vi "XP2i.vi"(4 "error in":T13, 7 "Command":T14) -> (0 "error out":T13, 3 "Response":T11)   [LabVIEW 2018]
uses:
  MOKO_LabViewLibrary/MokoLowLevel/MokoLowLovelControl/MLLC_Command.ctl
  MOKO_LabViewLibrary/MokoLowLevel/MokoLowLovelControl/MLLC_Error.ctl
  MOKO_LabViewLibrary/MokoLowLevel/MokoLowLovelControl/MLLC_Mode.ctl
  MOKO_LabViewLibrary/MokoLowLevel/MokoLowLovelControl/MLLC_Response.ctl
  MOKO_LabViewLibrary/MokoLowLevel/MokoLowLovelControl/MLLC_DriverName.ctl
  MOKO_LabViewLibrary/MokoLowLevel/MokoLowLovelControl/MLLC_ResponseInit.ctl
  MOKO_LabViewLibrary/MokoLowLevel/MokoLowLovelControl/MLLC_Request.ctl
  MOKO_LabViewLibrary/MokoLowLevel/MokoLowLovelControl/MLLC_ErrorCode.ctl
  MOKO_LabViewLibrary/MokoLowLevel/MokoLowLovelControl/MLLC_ConnectCluster.ctl
  MOKO_LabViewLibrary/MokoLowLevel/MokoLowLovelControl/MLLC_InterfaceType.ctl
  MOKO_LabViewLibrary/MokoLowLevel/MokoLowLovelControl/MLLC_OpenedSession.ctl
  MOKO_LabViewLibrary/MokoLowLevel/MokoLowLovelControl/MLLC_InterfaceSettings.ctl
  MOKO_LabViewLibrary/MokoLowLevel/MokoLowLovelControl/MLLC_InterfaceKind.ctl
  MOKO_LabViewLibrary/MokoLowLevel/MokoLowLovelControl/MLLC_Rs232Settings.ctl
panel:
  in  "Settings":T6={"Saved Data"=variant, "Permanent data"={"Connect"={"InterfaceType"=enum."VISA", "OpenedSession"="COM4", "InterfaceSettings"={"Interface"=enum."RS232", "EOS 4 read"=enum."Default (=EOS 4 write)", "EOS 4 write"=enum."CR (\\r)", "TMO, ms"=2000, "Sett"=variant(cluster{"Baud Rate":u32, "Data Bits":u16, "Parity":u16, "Stop Bits":u16, "Flow Control":u16, "Eho":bool} {"Baud Rate"=75, "Data Bits"=0, "Parity"=0, "Stop Bits"=0, "Flow Control"=0, "Eho"=FALSE})}}}}
  in  "Error Code":T7=5420
  in  "Request":T8="?MOD"
  in  "ResponseInit":T9="XP2I"
  in  "Driver Name":T10="Crystal XP2"
  in  "Mode":T12=enum."Check"
  # "XP2i"
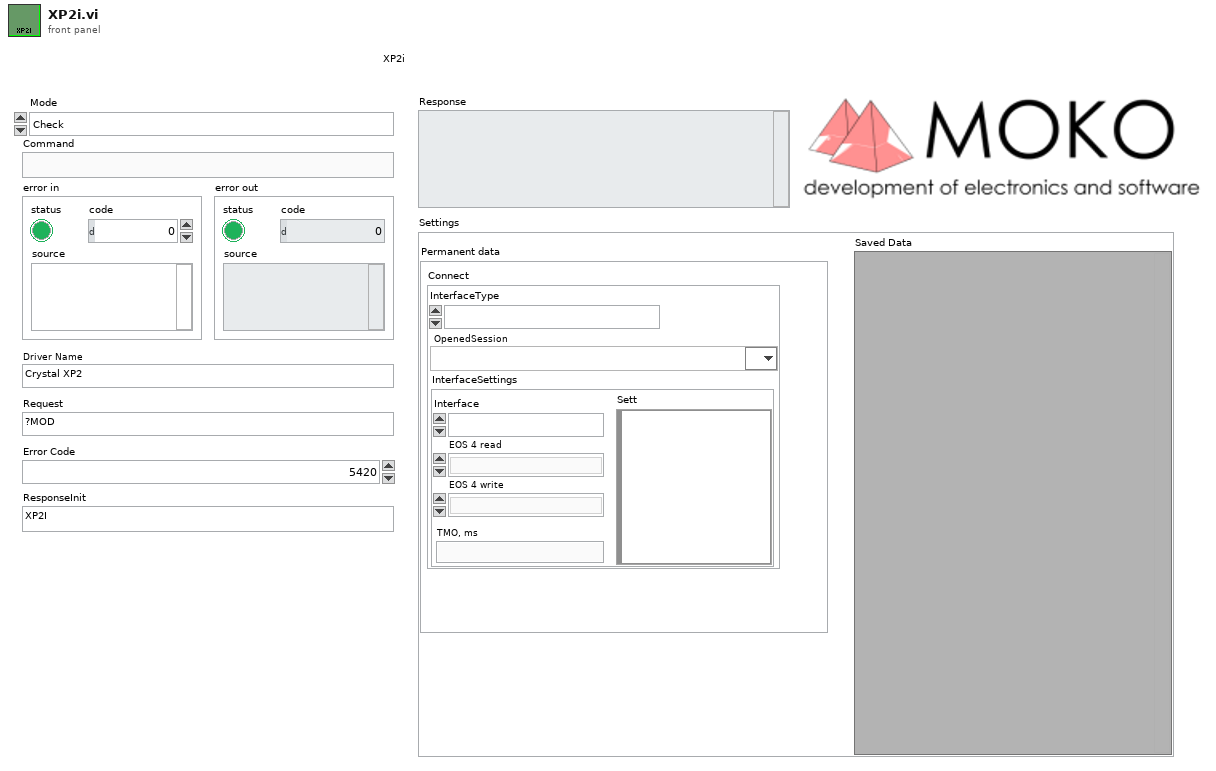
[diagram p1: front panel]
types:
  T1 = typedef "MLLC_ConnectCluster.ctl" = cluster{"InterfaceType":T2, "OpenedSession":T3, "InterfaceSettings":T4}
  T2 = typedef "MLLC_InterfaceType.ctl" = enum16{"VISA", "Prologix USB-GPIB"}
  T3 = typedef "MLLC_OpenedSession.ctl" = refnum<visa-resource-name>
  T4 = typedef "MLLC_InterfaceSettings.ctl" = cluster{"Interface":T5, "EOS 4 read":enum16{"Default (=EOS 4 write)", "CR (\\r)", "LF (\\n)", "None"}, "EOS 4 write":enum16{"CR+LF (\\r\\n)", "CR (\\r)", "LF (\\n)", "None"}, "TMO, ms":i32, "Sett":variant}
  T5 = typedef "MLLC_InterfaceKind.ctl" = enum16{"RS232", "GPIB", "USB", "Ethernet", "another"}
  T6 = cluster{"Saved Data":variant, "Permanent data":cluster{"Connect":T1}}
  T7 = typedef "MLLC_ErrorCode.ctl" = u32
  T8 = typedef "MLLC_Request.ctl" = string
  T9 = typedef "MLLC_ResponseInit.ctl" = string
  T10 = typedef "MLLC_DriverName.ctl" = string
  T11 = typedef "MLLC_Response.ctl" = string
  T12 = typedef "MLLC_Mode.ctl" = enum16{"get", "set", "close", "Init", "Check"}
  T13 = typedef "MLLC_Error.ctl" = errorcluster
  T14 = typedef "MLLC_Command.ctl" = string
  T15 = typedef "MLLC_Rs232Settings.ctl" = cluster{"Baud Rate":u32, "Data Bits":u16, "Parity":u16, "Stop Bits":u16, "Flow Control":u16, "Eho":bool, "Address":dbl}
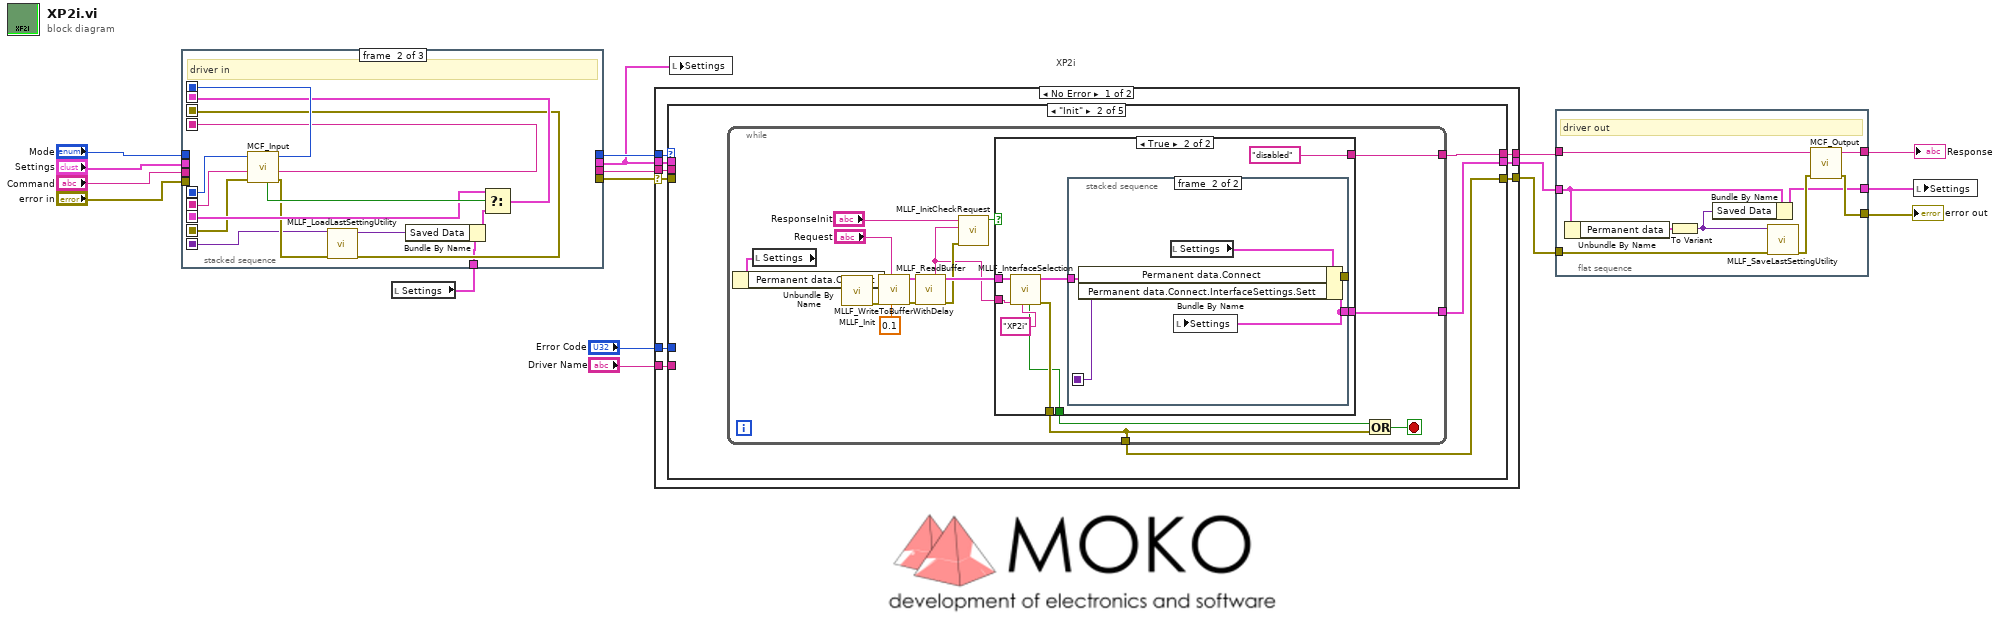
[diagram p0: block diagram]
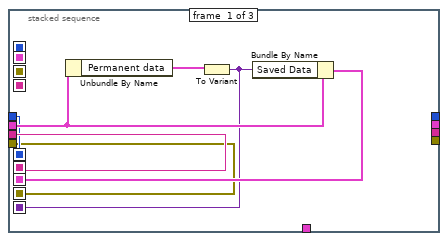
[diagram p2: hidden frame]
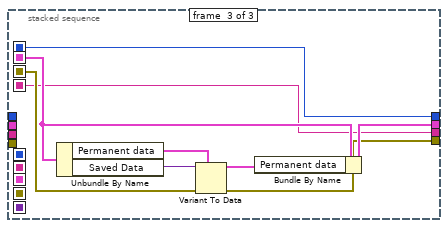
[diagram p3: hidden frame]
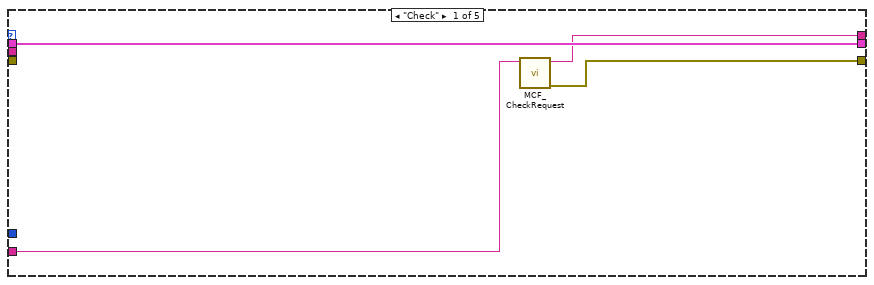
[diagram p4: hidden frame]
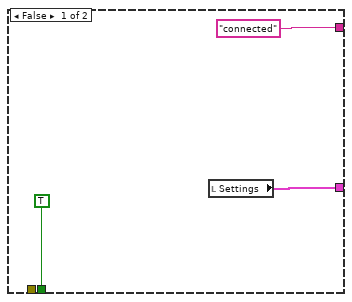
[diagram p5: hidden frame]
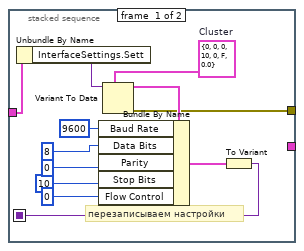
[diagram p6: hidden frame]
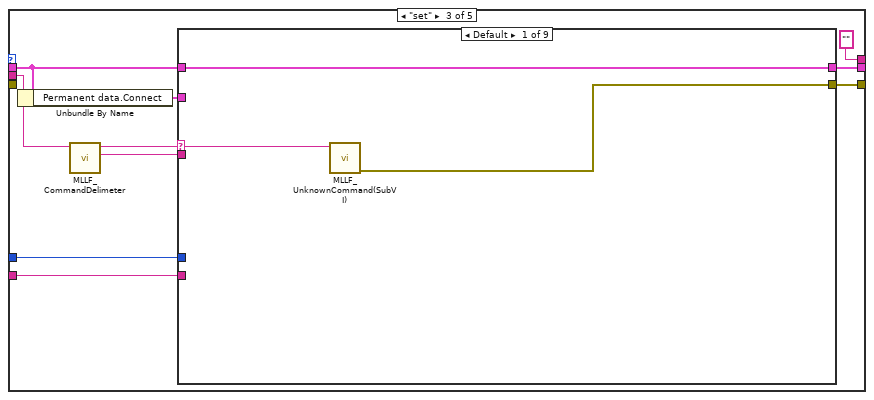
[diagram p7: hidden frame]
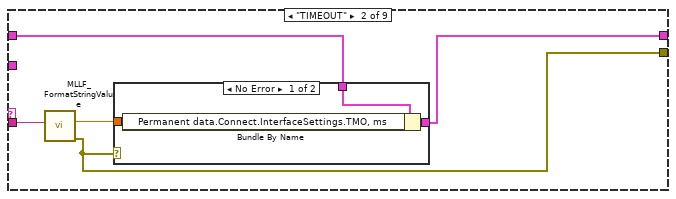
[diagram p8: hidden frame]
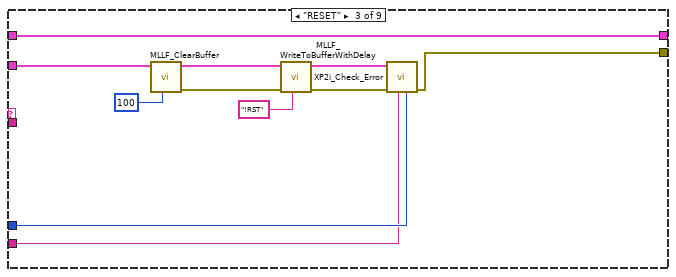
[diagram p10: hidden frame]
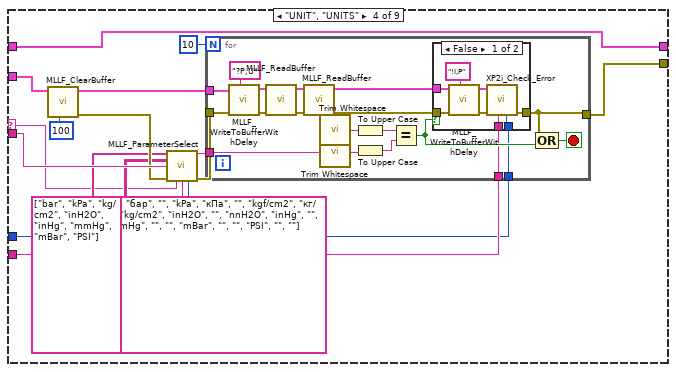
[diagram p11: hidden frame]
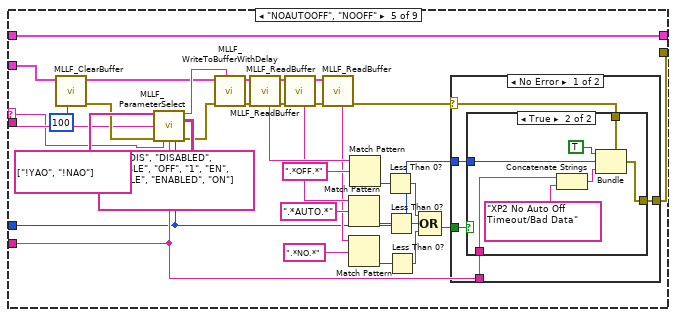
[diagram p13: hidden frame]
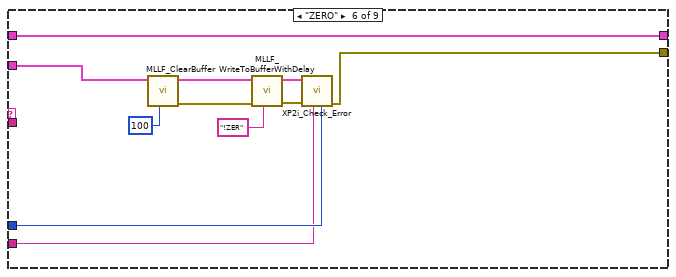
[diagram p16: hidden frame]
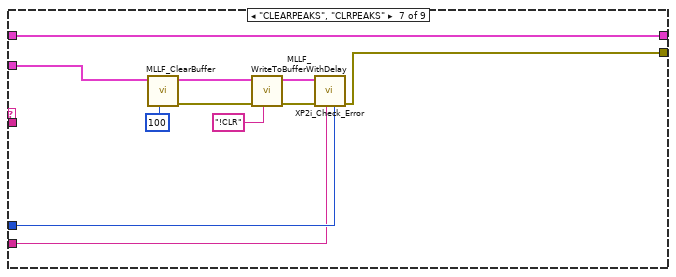
[diagram p17: hidden frame]
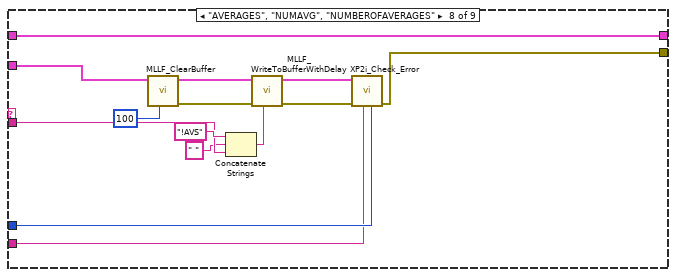
[diagram p18: hidden frame]
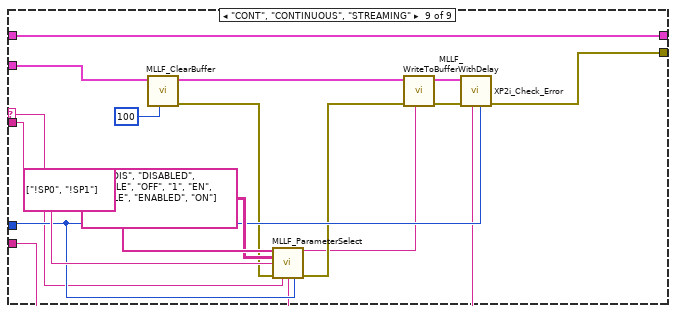
[diagram p19: hidden frame]
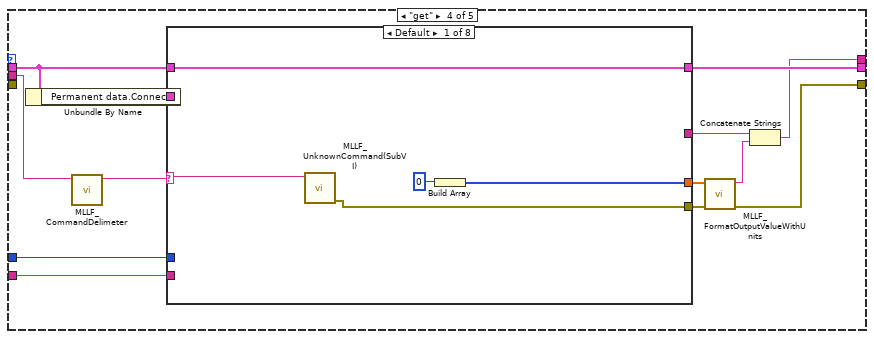
[diagram p20: hidden frame]
diagram:
  # "XP2i"
  n1 = local read "Settings"() -> (w7:T6)
  n2 = stacked-sequence {
    seq-local: [w20 _ _] -> [_ w36 _]
    seq-local: [w19 _ _] -> [_ w37 _]
    seq-local: [w22 _ _] -> [_ w32 _]
    seq-local: [w18 _ _] -> [_ w31 _]
    seq-local: [w21 _ _] -> [_ w27 _]
    seq-local: [_ w28 _] -> [_ _ w44]
    seq-local: [_ w38 _] -> [_ _ w41]
    seq-local: [_ w35 _] -> [_ _ w40]
    seq-local: [_ w34 _] -> [_ _ w45]
    tunnel: "Command" -> [w20 _ _]
    tunnel: "Mode" -> [w19 _ _]
    tunnel: "error in" -> [w18 _ _]
    tunnel: "Settings" -> [w23 _ _]
    tunnel: w7 -> [_ w26 _]
    tunnel: [_ _ w40] -> w9
    tunnel: [_ _ w43] -> w10
    tunnel: [_ _ w42] -> w8
    tunnel: [_ _ w41] -> w11
    frame #0 {
      n3 = Unbundle By Name(w23) -> ("Permanent data"=w24:cluster{"Connect":T1})
      n4 = To Variant(anything=w24) -> (Variant=w21:variant)
      n5 = Bundle By Name(cluster=w23, "Saved Data"=w21) -> (w22:T6)
    }
    frame #1 {
      # "driver in"
      n6 = call "MCF_Input.vi"("Error In"=w31, "Command in"=w36, "Mode in"=w37) -> ("Error Out"=w30:errorcluster, "Command out"=w35:string, "Mode out"=w38:T12, "Boolean"=w33:bool)  [unwired: 5 in]
      n7 = call "MLLF_LoadLastSettingUtility.vi"("Error In"=w30, "Save data in"=w27) -> ("Error Out"=w28:errorcluster, "Save data out"=w25:variant)  [unwired: 8 in]
      n8 = Bundle By Name(cluster=w26, "Saved Data"=w25) -> (w29:T6)
      n9 = Select(t=w32, s=w33, f=w29) -> (s? t:f=w34:T6)
    }
    frame #2 {
      n10 = Unbundle By Name(w45) -> ("Permanent data"=w46:cluster{"Connect":T1}, "Saved Data"=w39:variant)
      n11 = Variant To Data(error in=w44, type=w46, Variant=w39) -> (data=w47:cluster{"Connect":T1}, error out=w42:errorcluster)
      n12 = Bundle By Name(cluster=w45, "Permanent data"=w47) -> (w43:T6)
    }
  }
  n13 = case shown="No Error" w8 {
    selector: w8 -> [w53 w410]
    tunnel: [w48 w410] -> w4
    tunnel: w11 -> [w56 _]
    tunnel: [w55 _] -> w6
    tunnel: w9 -> [w54 _]
    tunnel: w10 -> [w50 w409]
    tunnel: "Error Code" -> [w52 _]
    tunnel: "Driver Name" -> [w51 _]
    tunnel: [w49 w409] -> w5
    frame No Error {
      n14 = case shown="\"Init\"" w56 {
        tunnel: [w58 w63 "" ("Output String") w294 "" ("Output String")] -> w55
        tunnel: w54 -> [_ _ w111 w287 _]
        tunnel: w53 -> [_ _ _ _ _]
        tunnel: w52 -> [_ _ w118 w297 _]
        tunnel: w51 -> [w59 _ w115 w296 _]
        tunnel: w50 -> [w60 _ w117 w298 w407]
        tunnel: [w60 w62 w116 w295 w407] -> w49
        tunnel: [w57 w61 w114 w288 w406] -> w48
        frame "Check" {
          n15 = call "MCF_CheckRequest.vi"("Driver Name"=w59) -> ("Error Out"=w57:errorcluster, "Output String"=w58:string)  [unwired: 9 in]
        }
        frame "Init" {
          n16 = while {
            tunnel: [w76] -> w61
            tunnel: [w73] -> w63
            tunnel: [w72] -> w62
            stop <- w78 stop-if-true
            n17 = local read "Settings"() -> (w67:T6)
            n18 = Unbundle By Name(w67) -> ("Permanent data.Connect"=w66:T1)
            n19 = call "MLLF_Init.vi"("DriverConnect in"=w66) -> ("Error Out"=w80:errorcluster, "DriverConnect out"=w79:T1)  [unwired: 7 in]
            n20 = call "MLLF_WriteToBufferWithDelay.vi"("Delay Time ( 0,05 s)"=0.1 ("Delay Time (s)"), "Command"="Request", "Error In"=w80, "DriverConnect in"=w79) -> ("Error Out"=w75:errorcluster, "DriverConnect out"=w65:T1)  [unwired: 6 in]
            n21 = call "MLLF_ReadBuffer.vi"("Error In"=w75, "DriverConnect in"=w65) -> ("Error Out"=w71:errorcluster, "DriverConnect out"=w81:T1, "String"=w64:string)  [unwired: 6 in]
            n22 = call "MLLF_InitCheckRequest.vi"("error in (no error)"=w71, "Answer"=w64, "Response Init"="ResponseInit") -> ("Design"=w70:bool)  [unwired: 5 in, 3 out]
            n23 = case shown="True" w70 {
              tunnel: w81 -> [_ w91]
              tunnel: [TRUE w87] -> w77
              tunnel: [_ w92] -> w76
              tunnel: ["connected" "disabled"] -> w73
              tunnel: [w82 w86] -> w72
              tunnel: w64 -> [_ w85]
              frame False {
                n24 = local read "Settings"() -> (w82:T6)
              }
              frame True {
                n25 = call "MLLF_InterfaceSelection.vi"("Driver Name"="XP2i" ("String"), "Answer:"=w85, "DriverConnect in"=w91) -> ("error out"=w92:T13, "DriverConnect out"=w90:T1, "stop init?"=w87:bool)  [unwired: 4 in, 2 out]
                n26 = stacked-sequence {
                  seq-local: [w96 _] -> [_ w105]
                  tunnel: w90 -> [w94 w106]
                  tunnel: [w97 _] -> _
                  tunnel: [_ w107] -> w86
                  frame #0 {
                    w98 = T15 {"Baud Rate"=0, "Data Bits"=0, "Parity"=0, "Stop Bits"=10, "Flow Control"=0, "Eho"=FALSE, "Address"=0.0}  # Cluster
                    # "перезаписываем настройки"
                    n27 = Unbundle By Name(w94) -> ("InterfaceSettings.Sett"=w93:variant)
                    n28 = Variant To Data(type=w98, Variant=w93) -> (data=w99:T15, error out=w97:errorcluster)  [unwired: 1 in]
                    n29 = Bundle By Name(cluster=w99, "Baud Rate"=u32 9600, "Data Bits"=u16 8 ("Serial Settings:Data Bits"), "Parity"=u16 0 ("Serial Settings:Parity"), "Stop Bits"=u16 10 ("Serial Settings:Stop Bits"), "Flow Control"=u16 0 ("Serial Settings:Flow Control")) -> (w104:T15)
                    n30 = To Variant(anything=w104) -> (Variant=w96:variant)
                  }
                  frame #1 {
                    n31 = local read "Settings"() -> (w108:T6)
                    n32 = Bundle By Name(cluster=w108, "Permanent data.Connect"=w106, "Permanent data.Connect.InterfaceSettings.Sett"=w105) -> (w107:T6)
                    n33 = local write "Settings"(w107) -> ()
                  }
                }
              }
            }
            n34 = Or(x=w77, y=w76) -> (x .or. y?=w78:bool)
          }
        }
        frame "set" {
          n35 = Unbundle By Name(w117) -> ("Permanent data.Connect"=w112:T1)
          n36 = call "MLLF_CommandDelimeter.vi"("command with param"=w111) -> ("param 1"=w109:string, "command"=w110:string)  [unwired: 6 in, 3 out]
          n37 = case shown="Default" w110 {
            selector: w110 -> [w120 _ _ w142 w186 _ _ _ w271]
            tunnel: w109 -> [_ w124 _ w154 w194 _ _ w261 w280]
            tunnel: w118 -> [_ _ w139 w152 w196 w239 w250 w265 w279]
            tunnel: w117 -> [w121 w125 w141 w145 w219 w244 w255 w269 w285]
            tunnel: [w121 w126 w141 w145 w219 w244 w255 w269 w285] -> w116
            tunnel: w115 -> [_ _ w138 w153 w197 w238 w249 w264 w270]
            tunnel: w112 -> [_ _ w132 w144 w188 w235 w246 w257 w273]
            tunnel: [w119 w122 w131 w143 w187 w234 w245 w256 w272] -> w114
            frame Default {
              n38 = call "MLLF_UnknownCommand(SubVI).vi"("Unknown command"=w120) -> ("error out"=w119:errorcluster)  [unwired: 10 in]
            }
            frame "TIMEOUT" {
              n39 = call "MLLF_FormatStringValue.vi"("String Value"=w124) -> ("error out"=w122:T13, "number"=w123:dbl)  [unwired: 8 in, 1 out]
              n40 = case shown="No Error" w122 {
                tunnel: [w129 w130] -> w126
                tunnel: w125 -> [w128 w130]
                tunnel: w123 -> [w127 _]
                frame No Error {
                  n41 = Bundle By Name(cluster=w128, "Permanent data.Connect.InterfaceSettings.TMO, ms"=w127) -> (w129:T6)
                }
                frame Error {
                }
              }
            }
            frame "RESET" {
              n42 = call "MLLF_ClearBuffer.vi"("Timeout(default = 300 ms)"=u32 100 ("Timeout"), "DriverConnect in"=w132) -> ("Error Out"=w136:errorcluster, "DriverConnect out"=w135:T1)  [unwired: 6 in, 1 out]
              n43 = call "MLLF_WriteToBufferWithDelay.vi"("Command"="!RST" ("String"), "Error In"=w136, "DriverConnect in"=w135) -> ("Error Out"=w134:errorcluster, "DriverConnect out"=w140:T1)  [unwired: 7 in]
              n44 = call "XP2i_Check_Error.vi"("Error Code"=w139, "Driver Name"=w138, "Error In"=w134, "DriverConnect in"=w140) -> ("Error Out"=w131:errorcluster)  [unwired: 6 in, 1 out]
            }
            frame "UNIT", "UNITS" {
              n45 = call "MLLF_ClearBuffer.vi"("Timeout(default = 300 ms)"=u32 100 ("Timeout"), "DriverConnect in"=w144) -> ("Error Out"=w151:errorcluster, "DriverConnect out"=w155:T1)  [unwired: 6 in, 1 out]
              n46 = call "MLLF_ParameterSelect.vi"("Command to equipment"=string[] ["bar", "kPa", "kg/cm2", "inH2O", "inHg", "mmHg", "mBar", "PSI"] ("Parameters 2 equipment"), "Names"=string[][] [["bar", "бар", ""], ["kPa", "кПа", ""], ["kgf/cm2", "кг/см2", "kg/cm2"], ["inH2O", "", "nnH2O"], ["inHg", "", ""], ["mmHg", "", ""], ["mBar", "", ""], ["PSI", "", ""]], "Input"=w154, "Error In"=w151, "Command"=w142, "Driver Name"=w153, "Error Code"=w152) -> ("Choice"=w149:string, "Error Out"=w150:errorcluster)  [unwired: 7 in]
              n47 = for {
                N: 10 -> [_]
                tunnel: w155 -> [w166]
                tunnel: [w160] -> w143
                tunnel: w149 -> [w164]
                tunnel: w153 -> [w158]
                tunnel: w152 -> [w157]
                tunnel: w150 -> [w165]
                stop <- w172 stop-if-true
                n48 = call "MLLF_WriteToBufferWithDelay.vi"("Command"="?P,U" ("String"), "Error In"=w165, "DriverConnect in"=w166) -> ("Error Out"=w168:errorcluster, "DriverConnect out"=w175:T1)  [unwired: 7 in]
                n49 = call "MLLF_ReadBuffer.vi"("Error In"=w168, "DriverConnect in"=w175) -> ("Error Out"=w171:errorcluster, "DriverConnect out"=w170:T1)  [unwired: 6 in, 1 out]
                n50 = call "MLLF_ReadBuffer.vi"("Error In"=w171, "DriverConnect in"=w170) -> ("Error Out"=w161:errorcluster, "DriverConnect out"=w162:T1, "String"=w169:string)  [unwired: 6 in]
                n51 = call <vilib>:"Trim Whitespace.vi"("string"=w169) -> ("trimmed string"=w167:string)  [unwired: 1 in]
                n52 = call <vilib>:"Trim Whitespace.vi"("string"=w164) -> ("trimmed string"=w163:string)  [unwired: 1 in]
                n53 = To Upper Case(1:w167) -> (0:w174:string)
                n54 = To Upper Case(1:w163) -> (0:w173:string)
                n55 = Equal?(x=w174, y=w173) -> (x = y?=w159:bool)
                n56 = case shown="False" w159 {
                  tunnel: w162 -> [w181 _]
                  tunnel: w161 -> [w180 w185]
                  tunnel: [w179 w185] -> w160
                  tunnel: w158 -> [w178 _]
                  tunnel: w157 -> [w177 _]
                  frame False {
                    n57 = call "MLLF_WriteToBufferWithDelay.vi"("Command"="!I,P" ("String"), "Error In"=w180, "DriverConnect in"=w181) -> ("Error Out"=w182:errorcluster, "DriverConnect out"=w183:T1)  [unwired: 7 in]
                    n58 = call "XP2i_Check_Error.vi"("Error Code"=w177, "Driver Name"=w178, "Error In"=w182, "DriverConnect in"=w183) -> ("Error Out"=w179:errorcluster)  [unwired: 6 in, 1 out]
                  }
                  frame True {
                  }
                }
                n59 = Compound Arithmetic op=OR(w160, w159) -> (w172:bool)
              }
            }
            frame "NOAUTOOFF", "NOOFF" {
              n60 = call "MLLF_ClearBuffer.vi"("Timeout(default = 300 ms)"=u32 100 ("Timeout"), "DriverConnect in"=w188) -> ("Error Out"=w195:errorcluster, "DriverConnect out"=w191:T1)  [unwired: 6 in, 1 out]
              n61 = call "MLLF_ParameterSelect.vi"("Command to equipment"=string[] ["!YAO", "!NAO"] ("Names"), "Names"=string[][] [["0", "DIS", "DISABLED", "DISABLE", "OFF"], ["1", "EN", "ENABLE", "ENABLED", "ON"]], "Input"=w194, "Error In"=w195, "Command"=w186, "Driver Name"=w197, "Error Code"=w196) -> ("Choice"=w193:string, "Error Out"=w192:errorcluster)  [unwired: 7 in]
              n62 = call "MLLF_WriteToBufferWithDelay.vi"("Command"=w193, "Error In"=w192, "DriverConnect in"=w191) -> ("Error Out"=w189:errorcluster, "DriverConnect out"=w218:T1)  [unwired: 7 in]
              n63 = call "MLLF_ReadBuffer.vi"("Error In"=w189, "DriverConnect in"=w218) -> ("Error Out"=w217:errorcluster, "DriverConnect out"=w216:T1, "String"=w204:string)  [unwired: 6 in]
              n64 = call "MLLF_ReadBuffer.vi"("Error In"=w217, "DriverConnect in"=w216) -> ("Error Out"=w215:errorcluster, "DriverConnect out"=w214:T1, "String"=w203:string)  [unwired: 6 in]
              n65 = call "MLLF_ReadBuffer.vi"("Error In"=w215, "DriverConnect in"=w214) -> ("Error Out"=w201:errorcluster, "String"=w202:string)  [unwired: 6 in, 1 out]
              n66 = Match Pattern(string=w203, regular expression=".*AUTO.*") -> (offset past match=w209:i32)  [unwired: 1 in, 3 out]
              n67 = Match Pattern(string=w202, regular expression=".*NO.*") -> (offset past match=w210:i32)  [unwired: 1 in, 3 out]
              n68 = Match Pattern(string=w204, regular expression=".*OFF.*") -> (offset past match=w208:i32)  [unwired: 1 in, 3 out]
              n69 = Less Than 0?(x=w208) -> (x < 0?=w211:bool)
              n70 = Less Than 0?(x=w209) -> (x < 0?=w212:bool)
              n71 = Less Than 0?(x=w210) -> (x < 0?=w213:bool)
              n72 = Compound Arithmetic op=OR(w211, w212, w213) -> (w200:bool)
              n73 = case shown="No Error" w201 {
                selector: w201 -> [w220 w233]
                tunnel: [w224 w233] -> w187
                tunnel: w200 -> [w223 _]
                tunnel: w196 -> [w222 _]
                tunnel: w197 -> [w221 _]
                frame No Error {
                  n74 = case shown="True" w223 {
                    tunnel: [w225 w231] -> w224
                    tunnel: w222 -> [_ w230]
                    tunnel: w221 -> [_ w228]
                    tunnel: w220 -> [w225 w226]
                    frame False {
                    }
                    frame True {
                      n75 = Concatenate Strings(w228, "XP2 No Auto Off Timeout/Bad Data") -> (w227:string)
                      n76 = Bundle(cluster=w226, "status"=TRUE, "code"=w230, "source"=w227) -> (w231:errorcluster)
                    }
                  }
                }
                frame Error {
                }
              }
            }
            frame "ZERO" {
              n77 = call "MLLF_ClearBuffer.vi"("Timeout(default = 300 ms)"=u32 100 ("Timeout"), "DriverConnect in"=w235) -> ("Error Out"=w242:errorcluster, "DriverConnect out"=w241:T1)  [unwired: 6 in, 1 out]
              n78 = call "MLLF_WriteToBufferWithDelay.vi"("Command"="!ZER" ("String"), "Error In"=w242, "DriverConnect in"=w241) -> ("Error Out"=w236:errorcluster, "DriverConnect out"=w240:T1)  [unwired: 7 in]
              n79 = call "XP2i_Check_Error.vi"("Error Code"=w239, "Driver Name"=w238, "Error In"=w236, "DriverConnect in"=w240) -> ("Error Out"=w234:errorcluster)  [unwired: 6 in, 1 out]
            }
            frame "CLEARPEAKS", "CLRPEAKS" {
              n80 = call "MLLF_ClearBuffer.vi"("Timeout(default = 300 ms)"=u32 100 ("Timeout"), "DriverConnect in"=w246) -> ("Error Out"=w253:errorcluster, "DriverConnect out"=w252:T1)  [unwired: 6 in, 1 out]
              n81 = call "MLLF_WriteToBufferWithDelay.vi"("Command"="!CLR" ("String"), "Error In"=w253, "DriverConnect in"=w252) -> ("Error Out"=w248:errorcluster, "DriverConnect out"=w251:T1)  [unwired: 7 in]
              n82 = call "XP2i_Check_Error.vi"("Error Code"=w250, "Driver Name"=w249, "Error In"=w248, "DriverConnect in"=w251) -> ("Error Out"=w245:errorcluster)  [unwired: 6 in, 1 out]
            }
            frame "AVERAGES", "NUMAVG", "NUMBEROFAVERAGES" {
              n83 = call "MLLF_ClearBuffer.vi"("Timeout(default = 300 ms)"=u32 100 ("Timeout"), "DriverConnect in"=w257) -> ("Error Out"=w268:errorcluster, "DriverConnect out"=w267:T1)  [unwired: 6 in, 1 out]
              n84 = Concatenate Strings("!AVS" ("String"), " " ("string"), w261) -> (w262:string)
              n85 = call "MLLF_WriteToBufferWithDelay.vi"("Command"=w262, "Error In"=w268, "DriverConnect in"=w267) -> ("Error Out"=w259:errorcluster, "DriverConnect out"=w266:T1)  [unwired: 7 in]
              n86 = call "XP2i_Check_Error.vi"("Error Code"=w265, "Driver Name"=w264, "Error In"=w259, "DriverConnect in"=w266) -> ("Error Out"=w256:errorcluster)  [unwired: 6 in, 1 out]
            }
            frame "CONT", "CONTINUOUS", "STREAMING" {
              n87 = call "MLLF_ClearBuffer.vi"("Timeout(default = 300 ms)"=u32 100 ("Timeout"), "DriverConnect in"=w273) -> ("Error Out"=w278:errorcluster, "DriverConnect out"=w284:T1)  [unwired: 6 in, 1 out]
              n88 = call "MLLF_ParameterSelect.vi"("Command to equipment"=string[] ["!SP0", "!SP1"] ("Names"), "Names"=string[][] [["0", "DIS", "DISABLED", "DISABLE", "OFF"], ["1", "EN", "ENABLE", "ENABLED", "ON"]], "Input"=w280, "Error In"=w278, "Command"=w271, "Driver Name"=w270, "Error Code"=w279) -> ("Choice"=w276:string, "Error Out"=w277:errorcluster)  [unwired: 7 in]
              n89 = call "MLLF_WriteToBufferWithDelay.vi"("Command"=w276, "Error In"=w277, "DriverConnect in"=w284) -> ("Error Out"=w275:errorcluster, "DriverConnect out"=w283:T1)  [unwired: 7 in]
              n90 = call "XP2i_Check_Error.vi"("Error Code"=w279, "Driver Name"=w270, "Error In"=w275, "DriverConnect in"=w283) -> ("Error Out"=w272:errorcluster)  [unwired: 6 in, 1 out]
            }
          }
        }
        frame "get" {
          n91 = Unbundle By Name(w298) -> ("Permanent data.Connect"=w289:T1)
          n92 = call "MLLF_CommandDelimeter.vi"("command with param"=w287) -> ("command"=w286:string)  [unwired: 6 in, 4 out]
          n93 = case shown="Default" w286 {
            selector: w286 -> [w300 _ _ _ _ _ _ _]
            tunnel: [w299 _ w315 w329 w346 w363 w380 w397] -> w293
            tunnel: w297 -> [_ _ _ _ _ _ _ _]
            tunnel: [w303 w306 w319 w336 w353 w370 w387 w404] -> w295
            tunnel: w298 -> [w303 w306 w319 w336 w353 w370 w387 w404]
            tunnel: [w301 w304 _ w333 w350 w367 w384 w401] -> w292
            tunnel: w296 -> [_ _ _ _ _ _ _ _]
            tunnel: [_ _ w310 _ _ _ _ _] -> w290
            tunnel: w289 -> [_ _ w307 w320 w337 w354 w371 w388]
            frame Default {
              n94 = call "MLLF_UnknownCommand(SubVI).vi"("Unknown command"=w300) -> ("error out"=w299:errorcluster)  [unwired: 10 in]
              n95 = Build Array(0 ("TimeOut")) -> (w301:i32[])
            }
            frame "TIMEOUT" {
              n96 = Unbundle By Name(w306) -> ("Permanent data.Connect.InterfaceSettings.TMO, ms"=w305:i32)
              n97 = Build Array(w305) -> (w304:i32[])
            }
            frame "PRESSURE" {
              n98 = call "MLLF_ClearBuffer.vi"("Timeout(default = 300 ms)"=u32 100 ("Timeout"), "DriverConnect in"=w307) -> ("Error Out"=w316:errorcluster, "DriverConnect out"=w317:T1)  [unwired: 6 in, 1 out]
              n99 = call "MLLF_WriteToBufferWithDelay.vi"("Command"="?PRE" ("String"), "Error In"=w316, "DriverConnect in"=w317) -> ("Error Out"=w309:errorcluster, "DriverConnect out"=w314:T1)  [unwired: 7 in]
              n100 = call "MLLF_ReadBuffer.vi"("Error In"=w309, "DriverConnect in"=w314) -> ("Error Out"=w315:errorcluster, "String"=w313:string)  [unwired: 6 in, 1 out]
              n101 = Match Pattern(string=w313, regular expression=",") -> (before substring=w311:string)  [unwired: 1 in, 3 out]
              n102 = call <vilib>:"Trim Whitespace.vi"("string"=w311) -> ("trimmed string"=w310:string)  [unwired: 1 in]
            }
            frame "PRESSUREHIGH" {
              n103 = call "MLLF_ClearBuffer.vi"("Timeout(default = 300 ms)"=u32 100 ("Timeout"), "DriverConnect in"=w320) -> ("Error Out"=w330:errorcluster, "DriverConnect out"=w331:T1)  [unwired: 6 in, 1 out]
              n104 = call "MLLF_WriteToBufferWithDelay.vi"("Command"="?P,H" ("String"), "Error In"=w330, "DriverConnect in"=w331) -> ("Error Out"=w322:errorcluster, "DriverConnect out"=w326:T1)  [unwired: 7 in]
              n105 = call "MLLF_ReadBuffer.vi"("Error In"=w322, "DriverConnect in"=w326) -> ("Error Out"=w325:errorcluster, "DriverConnect out"=w324:T1, "String"=w323:string)  [unwired: 6 in]
              n106 = call "MLLF_ReadBuffer.vi"("Error In"=w325, "DriverConnect in"=w324) -> ("Error Out"=w329:errorcluster)  [unwired: 6 in, 2 out]
              n107 = Match Pattern(string=w323, regular expression=",") -> (before substring=w327:string)  [unwired: 1 in, 3 out]
              n108 = Fract/Exp String To Number(use system decimal point (T)=FALSE, string=w327) -> (number=w334:dbl)  [unwired: 2 in, 1 out]
              n109 = Build Array(w334) -> (w333:dbl[])
            }
            frame "PRESSURELOW" {
              n110 = call "MLLF_ClearBuffer.vi"("Timeout(default = 300 ms)"=u32 100 ("Timeout"), "DriverConnect in"=w337) -> ("Error Out"=w347:errorcluster, "DriverConnect out"=w348:T1)  [unwired: 6 in, 1 out]
              n111 = call "MLLF_WriteToBufferWithDelay.vi"("Command"="?P,L" ("String"), "Error In"=w347, "DriverConnect in"=w348) -> ("Error Out"=w339:errorcluster, "DriverConnect out"=w343:T1)  [unwired: 7 in]
              n112 = call "MLLF_ReadBuffer.vi"("Error In"=w339, "DriverConnect in"=w343) -> ("Error Out"=w342:errorcluster, "DriverConnect out"=w341:T1, "String"=w340:string)  [unwired: 6 in]
              n113 = call "MLLF_ReadBuffer.vi"("Error In"=w342, "DriverConnect in"=w341) -> ("Error Out"=w346:errorcluster)  [unwired: 6 in, 2 out]
              n114 = Match Pattern(string=w340, regular expression=",") -> (before substring=w344:string)  [unwired: 1 in, 3 out]
              n115 = Fract/Exp String To Number(use system decimal point (T)=FALSE, string=w344) -> (number=w351:dbl)  [unwired: 2 in, 1 out]
              n116 = Build Array(w351) -> (w350:dbl[])
            }
            frame "AVERAGEPRESSURE", "AVGPRESS", "AVGPRESSURE" {
              n117 = call "MLLF_ClearBuffer.vi"("Timeout(default = 300 ms)"=u32 100 ("Timeout"), "DriverConnect in"=w354) -> ("Error Out"=w364:errorcluster, "DriverConnect out"=w365:T1)  [unwired: 6 in, 1 out]
              n118 = call "MLLF_WriteToBufferWithDelay.vi"("Command"="?P,A" ("String"), "Error In"=w364, "DriverConnect in"=w365) -> ("Error Out"=w356:errorcluster, "DriverConnect out"=w360:T1)  [unwired: 7 in]
              n119 = call "MLLF_ReadBuffer.vi"("Error In"=w356, "DriverConnect in"=w360) -> ("Error Out"=w359:errorcluster, "DriverConnect out"=w358:T1, "String"=w357:string)  [unwired: 6 in]
              n120 = call "MLLF_ReadBuffer.vi"("Error In"=w359, "DriverConnect in"=w358) -> ("Error Out"=w363:errorcluster)  [unwired: 6 in, 2 out]
              n121 = Match Pattern(string=w357, regular expression=",") -> (before substring=w361:string)  [unwired: 1 in, 3 out]
              n122 = Fract/Exp String To Number(use system decimal point (T)=FALSE, string=w361) -> (number=w368:dbl)  [unwired: 2 in, 1 out]
              n123 = Build Array(w368) -> (w367:dbl[])
            }
            frame "RANGE" {
              n124 = call "MLLF_ClearBuffer.vi"("Timeout(default = 300 ms)"=u32 100 ("Timeout"), "DriverConnect in"=w371) -> ("Error Out"=w381:errorcluster, "DriverConnect out"=w382:T1)  [unwired: 6 in, 1 out]
              n125 = call "MLLF_WriteToBufferWithDelay.vi"("Command"="?RNG" ("String"), "Error In"=w381, "DriverConnect in"=w382) -> ("Error Out"=w373:errorcluster, "DriverConnect out"=w377:T1)  [unwired: 7 in]
              n126 = call "MLLF_ReadBuffer.vi"("Error In"=w373, "DriverConnect in"=w377) -> ("Error Out"=w376:errorcluster, "DriverConnect out"=w375:T1, "String"=w374:string)  [unwired: 6 in]
              n127 = call "MLLF_ReadBuffer.vi"("Error In"=w376, "DriverConnect in"=w375) -> ("Error Out"=w380:errorcluster)  [unwired: 6 in, 2 out]
              n128 = Match Pattern(string=w374, regular expression=",") -> (before substring=w378:string)  [unwired: 1 in, 3 out]
              n129 = Fract/Exp String To Number(use system decimal point (T)=FALSE, string=w378) -> (number=w385:dbl)  [unwired: 2 in, 1 out]
              n130 = Build Array(w385) -> (w384:dbl[])
            }
            frame "ZERO" {
              n131 = call "MLLF_ClearBuffer.vi"("Timeout(default = 300 ms)"=u32 100 ("Timeout"), "DriverConnect in"=w388) -> ("Error Out"=w398:errorcluster, "DriverConnect out"=w399:T1)  [unwired: 6 in, 1 out]
              n132 = call "MLLF_WriteToBufferWithDelay.vi"("Command"="?Z,U" ("String"), "Error In"=w398, "DriverConnect in"=w399) -> ("Error Out"=w390:errorcluster, "DriverConnect out"=w394:T1)  [unwired: 7 in]
              n133 = call "MLLF_ReadBuffer.vi"("Error In"=w390, "DriverConnect in"=w394) -> ("Error Out"=w393:errorcluster, "DriverConnect out"=w392:T1, "String"=w391:string)  [unwired: 6 in]
              n134 = call "MLLF_ReadBuffer.vi"("Error In"=w393, "DriverConnect in"=w392) -> ("Error Out"=w397:errorcluster)  [unwired: 6 in, 2 out]
              n135 = Match Pattern(string=w391, regular expression=",") -> (before substring=w395:string)  [unwired: 1 in, 3 out]
              n136 = Fract/Exp String To Number(use system decimal point (T)=FALSE, string=w395) -> (number=w402:dbl)  [unwired: 2 in, 1 out]
              n137 = Build Array(w402) -> (w401:dbl[])
            }
          }
          n138 = call "MLLF_FormatOutputValueWithUnits.vi"("error in"=w293, "ValuesIn"=w292) -> ("error out"=w288:T13, "Result string"=w291:T14)  [unwired: 8 in]
          n139 = Concatenate Strings(w290, w291) -> (w294:string)
        }
        frame "close" {
          n140 = Unbundle By Name(w407) -> ("Permanent data.Connect.OpenedSession"=w408:T3)
          n141 = VISA Close(VISA resource name=w408) -> (error out=w406:errorcluster)  [unwired: 1 in]
        }
      }
    }
    frame Error {
    }
  }
  n142 = local write "Settings"(w10) -> ()
  n143 = flat-sequence {
    tunnel: [w419] -> w3
    tunnel: [w418] -> w1
    tunnel: w6 -> [w417]
    tunnel: w4 -> [w416]
    tunnel: w5 -> [w412]
    tunnel: [w414] -> w2
    frame #0 {
      # "driver out"
      n144 = Unbundle By Name(w412) -> ("Permanent data"=w411:cluster{"Connect":T1})
      n145 = To Variant(anything=w411) -> (Variant=w413:variant)
      n146 = Bundle By Name(cluster=w412, "Saved Data"=w413) -> (w414:T6)
      n147 = call "MLLF_SaveLastSettingUtility.vi"("error in"=w416, "Saved Data"=w413) -> ("error out"=w415:T13)  [unwired: 8 in, 1 out]
      n148 = call "MCF_Output.vi"("Error In"=w415, "Input"=w417) -> ("Error Out"=w418:errorcluster, "Output"=w419:string)  [unwired: 8 in]
    }
  }
  n149 = local write "Settings"(w2) -> ()
  "error out" <- w1
  "Response" <- w3
